vi "saveSettings2MCU.vi"(6 "error in (no error)":errorcluster, 7 "Starting Address":u16, 8 "Config":T1) -> (0 "error out":errorcluster)   [LabVIEW 2016]
uses:
  Settings/Settings.ctl
  Logging/Logging Configuration.ctl
  Hardware Configuration.ctl
  <vilib>/NI Modbus.llb/MB Serial Master Query Write Multiple Registers (poly).vi
  Acquisition.lvlib
  Logging/Logging.lvlib
  Settings/Settings.lvlib
panel:
  out "Exception Code":u8 format="%.0x"
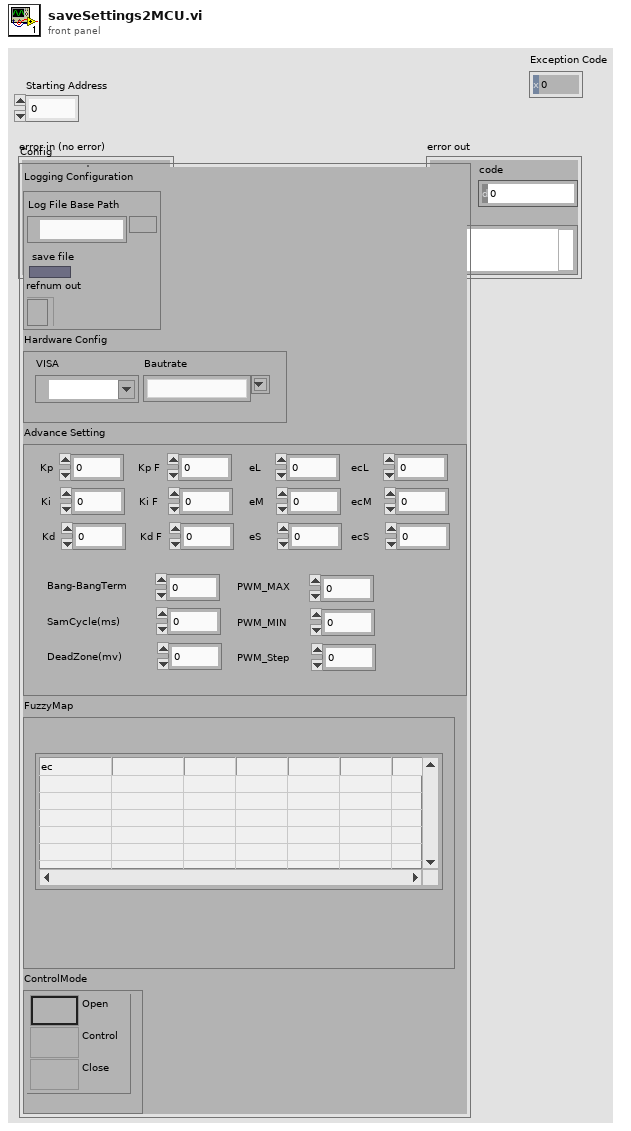
[diagram p1: front panel]
types:
  T1 = typedef "Settings.lvlib/Settings.ctl" = cluster{"Logging Configuration":T2, "Hardware Config":cluster{"Bautrate":string, "VISA":T3}, "Advance Setting":cluster{"PWM_Step":dbl, "PWM_MIN":dbl, "PWM_MAX":dbl, "DeadZone(mv)":dbl, "SamCycle(ms)":dbl, "Bang-BangTerm":dbl, "ecS":dbl, "ecM":dbl, "ecL":dbl, "eS":dbl, "eM":dbl, "eL":dbl, "Kd F":dbl, "Ki F":dbl, "Kp F":dbl, "Kd":dbl, "Ki":dbl, "Kp":dbl}, "FuzzyMap":cluster{"Table":string[][]}, "ControlMode":cluster{"Control":enum32{"1", "2", "4"}}}
  T2 = typedef "Logging.lvlib/Logging Configuration.ctl" = cluster{"Log File Base Path":path, "save file":bool, "refnum out":refnum<file>}
  T3 = typedef "Acquisition.lvlib/Hardware Configuration.ctl" = refnum<visa-resource-name>
  T4 = cluster{"PWM_Step":dbl, "PWM_MIN":dbl, "PWM_MAX":dbl, "DeadZone(mv)":dbl, "SamCycle(ms)":dbl, "Bang-BangTerm":dbl, "ecS":dbl, "ecM":dbl, "ecL":dbl, "eS":dbl, "eM":dbl, "eL":dbl, "Kd F":dbl, "Ki F":dbl, "Kp F":dbl, "Kd":dbl, "Ki":dbl, "Kp":dbl}
  T5 = cluster{"Mode":enum16{"RTU", "ASCII"}, "Slave Address":u8}
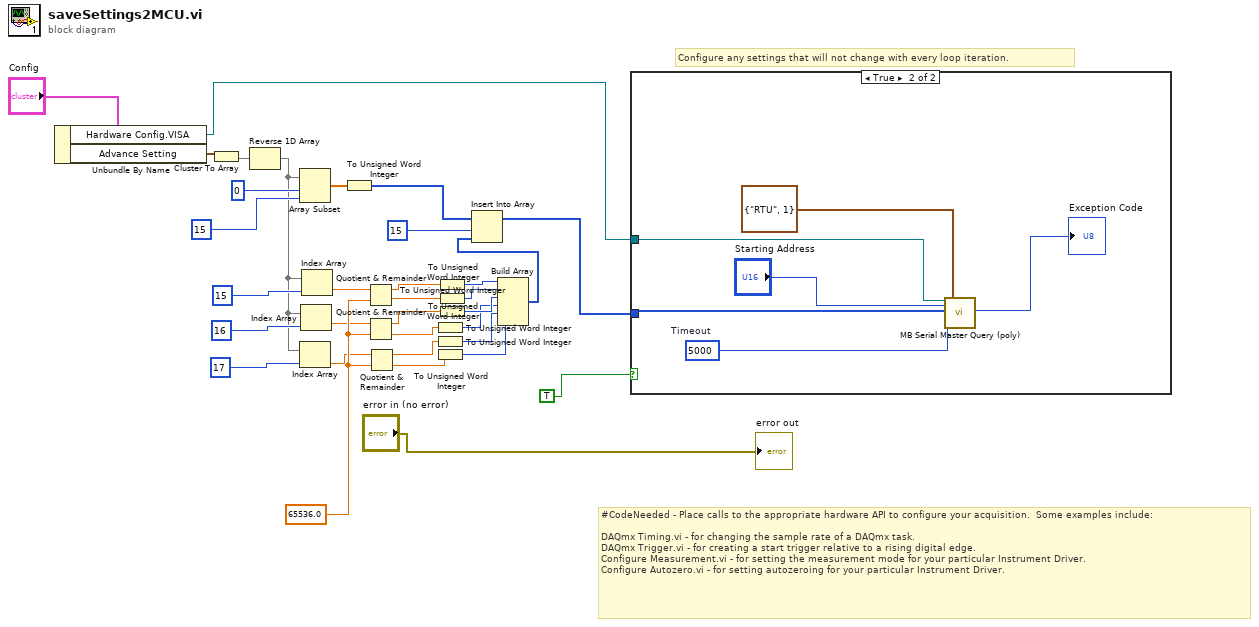
[diagram p0: block diagram]
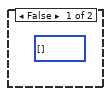
[diagram p2: hidden frame]
diagram:
  w13 = 65536.0 ("y")
  # "Configure any settings that will not change with every loop iteration."
  # "#CodeNeeded - Place calls to the appropriate hardware API to configure your acquisition.  Some examples include:\n\nDAQmx Timing.vi - for changing the sample rate of a DAQmx task.\nDAQmx Trigger.vi - for creating a start trigger relative to a rising digital edge.\nConfigure Measurement.vi - for setting the measurement mode for your particular Instrument Driver.\nConfigure Autozero.vi - for setting autozeroing for your particular Instrument Driver."
  n1 = Unbundle By Name("Config") -> ("Hardware Config.VISA"=w6:T3, "Advance Setting"=w5:T4)
  n2 = Cluster To Array(cluster=w5) -> (array=w4:dbl[])
  n3 = Reverse 1D Array(array=w4) -> (reversed array=w3:dbl[])
  n4 = Array Subset(array=w3, index=0, length=15) -> (w31:dbl[])
  n5 = Index Array(array=w3, index=17) -> (element=w12:dbl)
  n6 = Index Array(array=w3, index=16) -> (element=w11:dbl)
  n7 = Index Array(array=w3, index=15) -> (element=w23:dbl)
  n8 = To Unsigned Word Integer(number=w31) -> (unsigned 16bit integer=w26:u16[])
  n9 = Quotient & Remainder(x=w23, y=w13) -> (x-y*floor(x/y)=w24:dbl, floor(x/y)=w14:dbl)
  n10 = Quotient & Remainder(x=w11, y=w13) -> (x-y*floor(x/y)=w10:dbl, floor(x/y)=w9:dbl)
  n11 = Quotient & Remainder(x=w12, y=w13) -> (x-y*floor(x/y)=w8:dbl, floor(x/y)=w7:dbl)
  n12 = To Unsigned Word Integer(number=w9) -> (unsigned 16bit integer=w20:u16)
  n13 = To Unsigned Word Integer(number=w8) -> (unsigned 16bit integer=w19:u16)
  n14 = To Unsigned Word Integer(number=w7) -> (unsigned 16bit integer=w18:u16)
  n15 = To Unsigned Word Integer(number=w24) -> (unsigned 16bit integer=w25:u16)
  n16 = To Unsigned Word Integer(number=w14) -> (unsigned 16bit integer=w22:u16)
  n17 = To Unsigned Word Integer(number=w10) -> (unsigned 16bit integer=w21:u16)
  n18 = Build Array(w25, w22, w21, w20, w19, w18) -> (w17:u16[])
  n19 = Insert Into Array(array=w26, index=15, new element=w17) -> (w15:u16[])
  n20 = case shown="True" TRUE {
    tunnel: w6 -> [_ w39]
    tunnel: w15 -> [_ w34]
    frame False {
      (unwired) u16[] [] ("Input Registers")
    }
    frame True {
      w37 = u32 5000  # Timeout
      n21 = call-poly <vilib>:"MB Serial Master Query (poly).vi"("VISA resource name"=w39, "Starting Address"="Starting Address", "Registers"=w34, "Timeout"=w37, "Serial Parameters"=T5 {"Mode"=enum."RTU", "Slave Address"=1}) -> ("Exception Code"=→"Exception Code":u8)  [unwired: 12 in, 2 out]
    }
  }
  "error out" <- "error in (no error)"
